vi "replace classes.vi"   [LabVIEW 2013]
uses:
  <vilib>/Utility/traverseref.llb/TRef TravTarget.ctl
  source/table/data table.ctl
  <vilib>/Utility/traverseref.llb/VI Scripting - Traverse.lvlib
  source/table/data bus values.lvlib
types:
  T1 = typedef "TRef TravTarget.ctl" = enum16{"FP", "BD", "Other"}
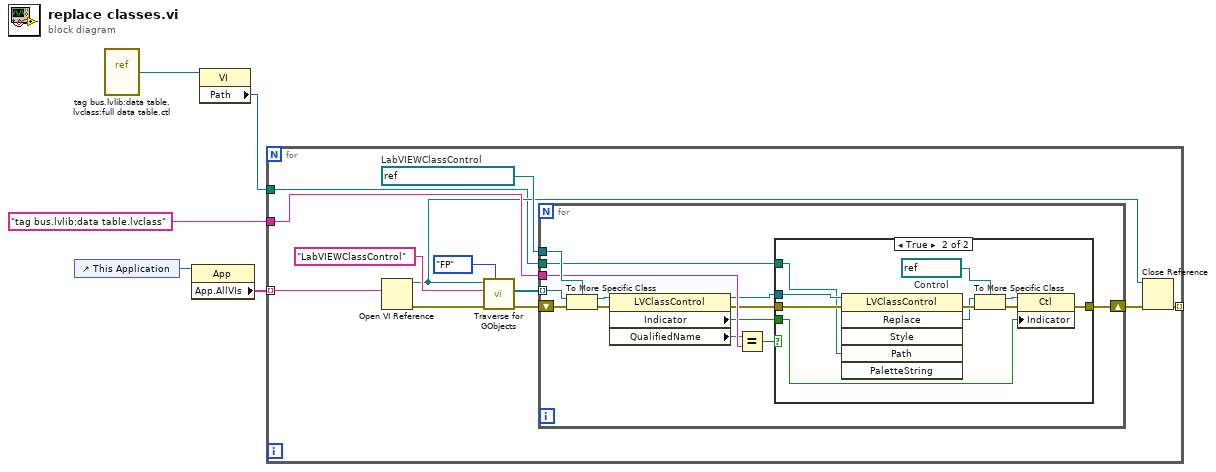
[diagram p0: block diagram]
diagram:
  n1 = control-ref of="This Application"() -> (w4:refnum<vi>)
  n2 = vi-ref "tag bus.lvlib:data table.lvclass:full data table.ctl"() -> (w3:refnum<vi>)
  n3 = property class="App"(reference=w4) -> ("App.AllVIs"=w5:string[])  [unwired: 1 in, 2 out]
  n4 = property class="VI"(reference=w3) -> ("Path"=w2:path)  [unwired: 1 in, 2 out]
  n5 = for {
    tunnel: w5 -> [w17] mode=indexing
    tunnel: "tag bus.lvlib:data table.lvclass" ("class name") -> [w10]
    tunnel: w2 -> [w7]
    tunnel: [w6] -> _ mode=indexing
    w11 = refnum<vi> refnum  # LabVIEWClassControl
    n6 = Open VI Reference(vi path=w17) -> (vi reference=w9:refnum<vi>, error out=w16:errorcluster)  [unwired: 5 in]
    n7 = call <vilib>:"Traverse for GObjects.vi"("Traverse Target"=TRef_TravTarget."FP", "error in (no error)"=w16, "Class Name"="LabVIEWClassControl", "VI Refnum"=w9) -> ("error out"=w12:errorcluster, "References"=w13:refnum<vi>[])  [unwired: 4 in, 2 out]
    n8 = for {
      tunnel: w13 -> [w29] mode=indexing
      shift-right: [w19] -> w8
      shift-left: w12 -> [w30]
      tunnel: w11 -> [w28]
      tunnel: w10 -> [w25]
      tunnel: w7 -> [w18]
      n9 = To More Specific Class(target class=w28, reference=w29, error in=w30) -> (specific class reference=w27:refnum<vi>, error out=w26:errorcluster)
      n10 = property class="LVClassControl"(reference=w27, error in=w26) -> (reference out=w21:refnum<vi>, error out=w20:errorcluster, "Indicator"=w22:bool, "QualifiedName"=w24:string)
      n11 = Equal?(x=w24, y=w25) -> (x = y?=w23:bool)
      n12 = case shown="True" w23 {
        tunnel: w22 -> [_ w32]
        tunnel: w21 -> [_ w40]
        tunnel: w20 -> [w31 w41]
        tunnel: [w31 w37] -> w19
        tunnel: w18 -> [_ w39]
        frame False {
        }
        frame True {
          w33 = refnum<vi> refnum  # Control
          n13 = invoke class="LVClassControl" method="Replace"(reference=w40, error in=w41, "Path"=w39) -> (error out=w38:errorcluster, "Replace"=w35:refnum<vi>)  [unwired: 3 in, 4 out]
          n14 = To More Specific Class(target class=w33, reference=w35, error in=w38) -> (specific class reference=w34:refnum<vi>, error out=w36:errorcluster)
          n15 = property class="Ctl"(reference=w34, error in=w36, "Indicator"=w32) -> (error out=w37:errorcluster)  [unwired: 1 out]
        }
      }
    }
    n16 = Close Reference(reference=w9, error in (no error)=w8) -> (error out=w6:errorcluster)
  }
